vi "Connect.vi"(8 "error in (no error)":errorcluster, 9 "Serial Config":T1 {"Parity" items=["None", "Odd", "Even"]; "Flow Ctl" items=["None"]; "Baud" items=["4800"=4800, "9600"=9600, "19200"=19200, "38400"=38400]}, 11 "B&K Precision 9120 series in":refnum<class "B&K Precision 9120 series.lvclass">) -> (0 "error out":errorcluster, 1 "result":string, 3 "B&K Precision 9120 series out":refnum<class "B&K Precision 9120 series.lvclass">)   [LabVIEW 2014, in "B&K Precision 9120 series.lvclass"]
uses:
  B&K Precision 9120 series.lvclass
  Serial_Config.ctl
  B&K Precision 9120 series.lvclass/B&K Precision 9120 series.ctl
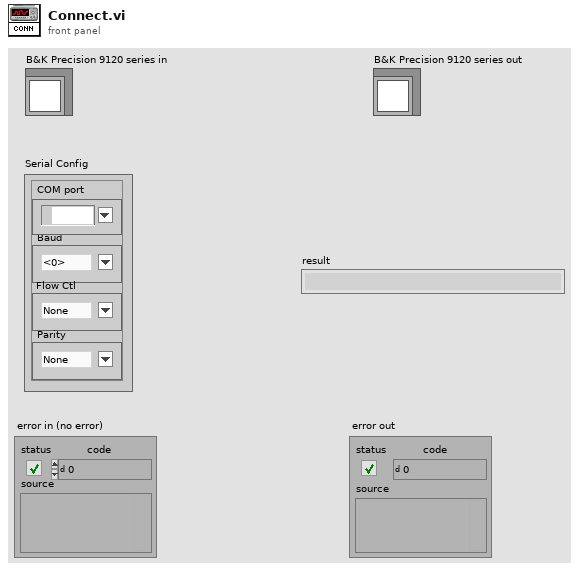
[diagram p1: front panel]
types:
  T1 = typedef "B&K Precision 9120 series.lvclass/Serial_Config.ctl" = cluster{"Baud":u32, "Flow Ctl":u16, "COM port":refnum<visa-resource-name>, "Parity":u16}
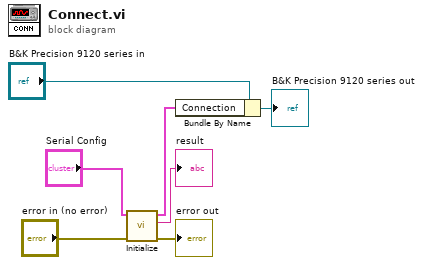
[diagram p0: block diagram]
diagram:
  n1 = call "Initialize.vi"("Connection in"="Serial Config", "error in (no error)"="error in (no error)") -> ("Connection out"=w1:T1, "read buffer"=→"result":string, "error out"=→"error out":errorcluster)  [unwired: 6 in]
  n2 = Bundle By Name(cluster="B&K Precision 9120 series in", "Connection"=w1) -> (→"B&K Precision 9120 series out":refnum<class "B&K Precision 9120 series.lvclass">)
